vi "Service Mode Version Parse LE.vi"(0 "GEA2 Reference In":refnum<k24>, 5 "Version Selection":T1, 11 "Error In":errorcluster) -> (1 "Crit 1":string, 2 "Crit 2":string, 3 "Crit 3":string, 4 "GEA2 Reference Out":refnum<k24>, 6 "NonCrit 2":string, 8 "NonCrit 3":string, 10 "NonCrit 4":string, 12 "Crit 4":string, 13 "NonCrit 1":string, 15 "Error Out":errorcluster)   [LabVIEW 2016, in "TLMB.lvlib"]
uses:
  Projects/TLMB.lvlib
  Q:/Common/DLLs/GEA3/GeaCommunication.dll
  Common/DLLs/GEA3/GeaCommunication.dll
  type defs/Service Mode Version Selection.ctl
  Common/LabVIEW GEA2 Toolkit/LabVIEW_GEA2_Toolkit.lvlibp/type defs/Source_Destination.ctl
  Common/LabVIEW GEA2 Toolkit/LabVIEW_GEA2_Toolkit.lvlibp/type defs/ERD Read Data In.ctl
  Common/LabVIEW GEA2 Toolkit/LabVIEW_GEA2_Toolkit.lvlibp/type defs/Data Type.ctl
  Common/LabVIEW GEA2 Toolkit/LabVIEW_GEA2_Toolkit.lvlibp
panel:
  in  "Standalone?":bool
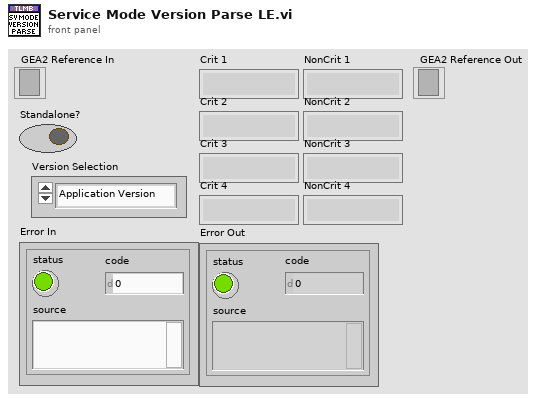
[diagram p1: front panel]
types:
  T1 = typedef "TLMB.lvlib/Service Mode Version Selection.ctl" = enum16{"Application Version", "XML Version"}
  T2 = typedef "LabVIEW_GEA2_Toolkit.lvlibp/Source_Destination.ctl" = cluster{"Source":u8, "Destination":u8}
  T3 = typedef "LabVIEW_GEA2_Toolkit.lvlibp/ERD Read Data In.ctl" = cluster{"ERD Number":u16, "Data Type":T4}
  T4 = typedef "LabVIEW_GEA2_Toolkit.lvlibp/Data Type.ctl" = enum16{"string", "boolean", "uint8_t", "uint16_t", "uint32_t", "uint64_t", "int8_t", "int16_t", "int32_t", "int64_t"}
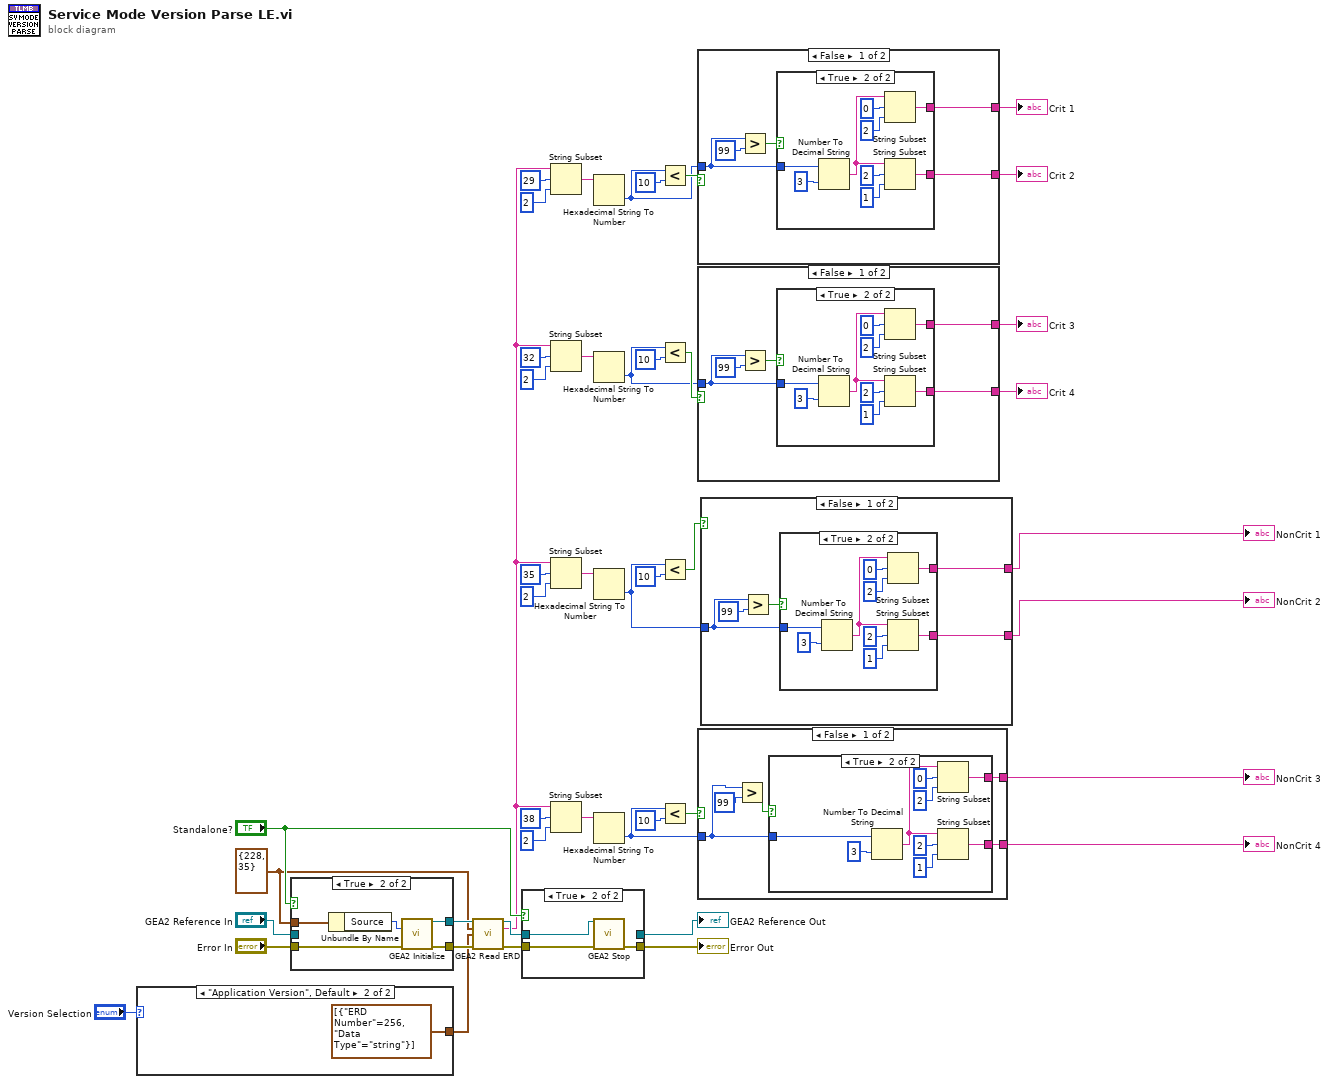
[diagram p0: block diagram]
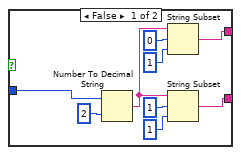
[diagram p2: hidden frame]
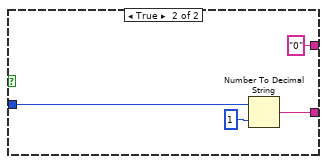
[diagram p3: hidden frame]
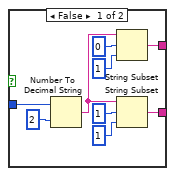
[diagram p4: hidden frame]
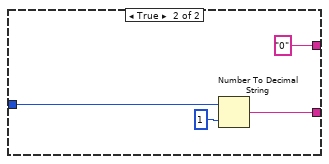
[diagram p5: hidden frame]
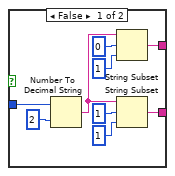
[diagram p6: hidden frame]
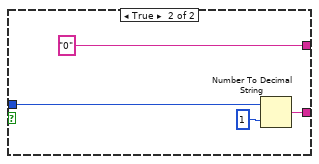
[diagram p7: hidden frame]
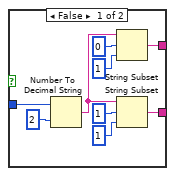
[diagram p8: hidden frame]
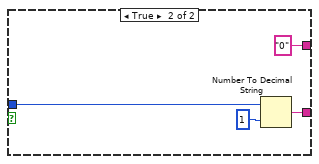
[diagram p9: hidden frame]
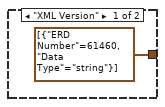
[diagram p10: hidden frame]
diagram:
  w37 = T2 {"Source"=228, "Destination"=35} ("GEA Inputs")
  n1 = case shown="\"Application Version\", Default" "Version Selection" {
    tunnel: [T3[] [{"ERD Number"=61460, "Data Type"=enum."string"}] ("Read ERD List") T3[] [{"ERD Number"=256, "Data Type"=enum."string"}] ("Read ERD List")] -> w35
    frame "XML Version" {
    }
    frame "Application Version", Default {
    }
  }
  n2 = case shown="True" "Standalone?" {
    tunnel: "Error In" -> [w48 w54]
    tunnel: [w48 w53] -> w40
    tunnel: "GEA2 Reference In" -> [w49 _]
    tunnel: [w49 w52] -> w38
    tunnel: w37 -> [_ w50]
    frame False {
    }
    frame True {
      n3 = Unbundle By Name(w50) -> ("Source"=w51:u8)
      n4 = call "GEA2 Initialize.vi"("Source Address"=w51, "error in"=w54) -> ("GEA2 Reference Out"=w52:refnum<k24>, "error out"=w53:errorcluster)  [unwired: 11 in, 1 out]
    }
  }
  n5 = call "GEA2 Read ERD.vi"("GEA2 Reference In"=w38, "GEA Inputs"=w37, "Read ERD List"=w35, "Error In"=w40) -> ("GEA2 Reference Out"=w36:refnum<k24>, "Raw Data Out"=w25:string, "Error Out"=w39:errorcluster)  [unwired: 8 in, 1 out]
  n6 = case shown="True" "Standalone?" {
    tunnel: [w55 w59] -> w43
    tunnel: w36 -> [w56 w58]
    tunnel: [w56 _] -> w42
    tunnel: w39 -> [w55 w57]
    frame False {
    }
    frame True {
      n7 = call "GEA2 Stop.vi"("GEA2 Reference In"=w58, "Error In"=w57) -> ("Error Out"=w59:errorcluster)  [unwired: 13 in]
    }
  }
  "Error Out" <- w43
  "GEA2 Reference Out" <- w42
  n8 = String Subset(string=w25, offset (0)=29, length (rest)=2 ("length (rest)")) -> (substring=w24:string)
  n9 = String Subset(string=w25, offset (0)=32, length (rest)=2 ("length (rest)")) -> (substring=w23:string)
  n10 = String Subset(string=w25, offset (0)=35, length (rest)=2 ("length (rest)")) -> (substring=w22:string)
  n11 = String Subset(string=w25, offset (0)=38, length (rest)=2 ("length (rest)")) -> (substring=w21:string)
  n12 = Hexadecimal String To Number(string=w24) -> (number=w16:u32)  [unwired: 2 in, 1 out]
  n13 = Hexadecimal String To Number(string=w23) -> (number=w11:u32)  [unwired: 2 in, 1 out]
  n14 = Hexadecimal String To Number(string=w22) -> (number=w2:u32)  [unwired: 2 in, 1 out]
  n15 = Hexadecimal String To Number(string=w21) -> (number=w1:u32)  [unwired: 2 in, 1 out]
  n16 = Less?(x=w16, y=u32 10) -> (x < y?=w19:bool)
  n17 = Less?(x=w11, y=u32 10) -> (x < y?=w12:bool)
  n18 = Less?(x=w2, y=u32 10) -> (x < y?=w7:bool)
  n19 = Less?(x=w1, y=u32 10) -> (x < y?=w6:bool)
  n20 = case shown="False" w19 {
    tunnel: [w64 "0"] -> w17
    tunnel: w16 -> [w62 w84]
    tunnel: [w63 w83] -> w18
    frame False {
      n21 = Greater?(x=w62, y=u32 99) -> (0:w60:bool)
      n22 = case shown="True" w60 {
        tunnel: [w67 w78] -> w64
        tunnel: [w66 w77] -> w63
        tunnel: w62 -> [w68 w74]
        frame False {
          n23 = Number To Decimal String(number=w68, width (-)=i16 2) -> (decimal integer string=w73:string)
          n24 = String Subset(string=w73, offset (0)=0, length (rest)=1 ("length (rest)")) -> (substring=w67:string)
          n25 = String Subset(string=w73, offset (0)=1, length (rest)=1 ("length (rest)")) -> (substring=w66:string)
        }
        frame True {
          n26 = Number To Decimal String(number=w74, width (-)=i16 3) -> (decimal integer string=w81:string)
          n27 = String Subset(string=w81, offset (0)=0, length (rest)=2 ("length (rest)")) -> (substring=w78:string)
          n28 = String Subset(string=w81, offset (0)=2, length (rest)=1 ("length (rest)")) -> (substring=w77:string)
        }
      }
    }
    frame True {
      n29 = Number To Decimal String(number=w84, width (-)=i16 1) -> (decimal integer string=w83:string)
    }
  }
  "Crit 1" <- w17
  "Crit 2" <- w18
  n30 = case shown="False" w12 {
    tunnel: [w91 "0"] -> w15
    tunnel: w11 -> [w89 w111]
    tunnel: [w90 w110] -> w14
    frame False {
      n31 = Greater?(x=w89, y=u32 99) -> (0:w87:bool)
      n32 = case shown="True" w87 {
        tunnel: [w93 w105] -> w91
        tunnel: [w92 w104] -> w90
        tunnel: w89 -> [w94 w101]
        frame False {
          n33 = Number To Decimal String(number=w94, width (-)=i16 2) -> (decimal integer string=w100:string)
          n34 = String Subset(string=w100, offset (0)=0, length (rest)=1 ("length (rest)")) -> (substring=w93:string)
          n35 = String Subset(string=w100, offset (0)=1, length (rest)=1 ("length (rest)")) -> (substring=w92:string)
        }
        frame True {
          n36 = Number To Decimal String(number=w101, width (-)=i16 3) -> (decimal integer string=w108:string)
          n37 = String Subset(string=w108, offset (0)=0, length (rest)=2 ("length (rest)")) -> (substring=w105:string)
          n38 = String Subset(string=w108, offset (0)=2, length (rest)=1 ("length (rest)")) -> (substring=w104:string)
        }
      }
    }
    frame True {
      n39 = Number To Decimal String(number=w111, width (-)=i16 1) -> (decimal integer string=w110:string)
    }
  }
  "Crit 3" <- w15
  "Crit 4" <- w14
  n40 = case shown="False" w6 {
    tunnel: [w118 "0"] -> w3
    tunnel: w1 -> [w115 w138]
    tunnel: [w117 w137] -> w4
    frame False {
      n41 = Greater?(x=w115, y=u32 99) -> (0:w116:bool)
      n42 = case shown="True" w116 {
        tunnel: w115 -> [w119 w135]
        tunnel: [w121 w131] -> w118
        tunnel: [w120 w130] -> w117
        frame False {
          n43 = Number To Decimal String(number=w119, width (-)=i16 2) -> (decimal integer string=w122:string)
          n44 = String Subset(string=w122, offset (0)=0, length (rest)=1 ("length (rest)")) -> (substring=w121:string)
          n45 = String Subset(string=w122, offset (0)=1, length (rest)=1 ("length (rest)")) -> (substring=w120:string)
        }
        frame True {
          n46 = Number To Decimal String(number=w135, width (-)=i16 3) -> (decimal integer string=w134:string)
          n47 = String Subset(string=w134, offset (0)=0, length (rest)=2 ("length (rest)")) -> (substring=w131:string)
          n48 = String Subset(string=w134, offset (0)=2, length (rest)=1 ("length (rest)")) -> (substring=w130:string)
        }
      }
    }
    frame True {
      n49 = Number To Decimal String(number=w138, width (-)=i16 1) -> (decimal integer string=w137:string)
    }
  }
  "NonCrit 3" <- w3
  "NonCrit 4" <- w4
  n50 = case shown="False" w7 {
    tunnel: [w145 "0"] -> w10
    tunnel: w2 -> [w142 w165]
    tunnel: [w144 w164] -> w9
    frame False {
      n51 = Greater?(x=w142, y=u32 99) -> (0:w143:bool)
      n52 = case shown="True" w143 {
        tunnel: w142 -> [w147 w162]
        tunnel: [w149 w158] -> w145
        tunnel: [w146 w157] -> w144
        frame False {
          n53 = Number To Decimal String(number=w147, width (-)=i16 2) -> (decimal integer string=w148:string)
          n54 = String Subset(string=w148, offset (0)=0, length (rest)=1 ("length (rest)")) -> (substring=w149:string)
          n55 = String Subset(string=w148, offset (0)=1, length (rest)=1 ("length (rest)")) -> (substring=w146:string)
        }
        frame True {
          n56 = Number To Decimal String(number=w162, width (-)=i16 3) -> (decimal integer string=w161:string)
          n57 = String Subset(string=w161, offset (0)=0, length (rest)=2 ("length (rest)")) -> (substring=w158:string)
          n58 = String Subset(string=w161, offset (0)=2, length (rest)=1 ("length (rest)")) -> (substring=w157:string)
        }
      }
    }
    frame True {
      n59 = Number To Decimal String(number=w165, width (-)=i16 1) -> (decimal integer string=w164:string)
    }
  }
  "NonCrit 1" <- w10
  "NonCrit 2" <- w9
